vi "Find Vireo Device Id.vi"(10 "error in (no error)":errorcluster, 11 "XML in":refnum<k20>) -> (2 "error out":errorcluster, 3 "XML":refnum<k20>, 5 "Vireo Target ID":string)   [LabVIEW 2020, in "PicoG-Processor.lvlib" / "WebProjectWatcher.lvclass"]
uses:
  WebProjectWatcher.lvclass
  <vilib>/xml/Close Reference(Node).vi
  <vilib>/xml/NI_XML.lvlib
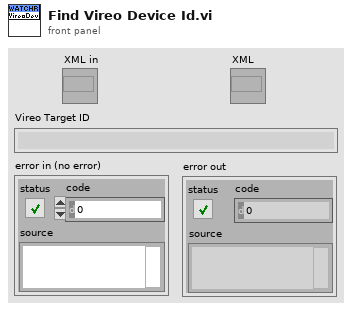
[diagram p1: front panel]
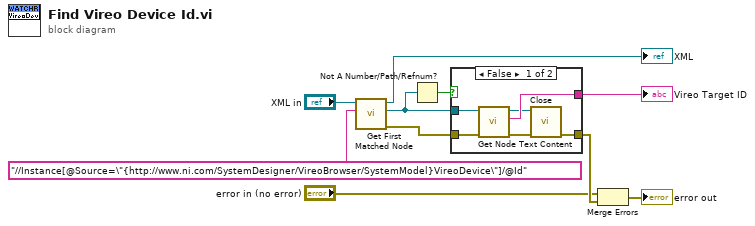
[diagram p0: block diagram]
diagram:
  n1 = call <vilib>:"Get First Matched Node.vi"("XPath expression"="//Instance[@Source=\"{http://www.ni.com/SystemDesigner/VireoBrowser/SystemModel}VireoDevice\"]/@Id", "node in"="XML in") -> ("error out"=w9:errorcluster, "node result"=w5:refnum<k20>, "node out"=→"XML":refnum<k20>)  [unwired: 7 in]
  n2 = Not A Number/Path/Refnum?(number/path/refnum=w5) -> (NaN/Path/Refnum?=w4:bool)
  n3 = case shown="False" w4 {
    tunnel: w9 -> [w16 w17]
    tunnel: [w15 _] -> w7
    tunnel: w5 -> [w12 _]
    tunnel: [w11 w17] -> w3
    frame False {
      n4 = call <vilib>:"Get Node Text Content.vi"("error in (no error)"=w16, "node in"=w12) -> ("error out"=w13:errorcluster, "node text"=w15:string, "node out"=w14:refnum<k20>)  [unwired: 7 in]
      n5 = call-poly <vilib>:"Close.vi"("error in (no error)"=w13, "node"=w14) -> ("error out"=w11:errorcluster)  [unwired: 7 in]
    }
    frame True {
    }
  }
  "Vireo Target ID" <- w7
  n6 = Merge Errors("error in (no error)", w3) -> (→"error out":errorcluster)
